vi "Fetch Cal Standard.vi"(0 "NICal5501 in":refnum<class "Cal Standard.lvclass">, 11 "error in":errorcluster) -> (4 "NICal5501 out":refnum<class "Cal Standard.lvclass">, 15 "error out":errorcluster)   [LabVIEW 2023, in "NI Cal-5501 Cal Standard.lvlib" / "Cal Standard.lvclass"]
uses:
  Cal Standard.lvclass
  C:/srd-semi-rfcal-software/AuxTools/STSRFFixtureCharactUtility/Source/Code Modules/Fixture/Instruments/Cal Standard/Cal Standard Base/Cal Standard Base.lvclass
  Cal Standard.lvclass/Cal Standard.ctl
  Instruments/Cal Standard/Type Definitions/One-Port Cal Standard.ctl
  Instruments/Cal Standard/Type Definitions/One-Port Charact Data.ctl
  Instruments/Cal Standard/Type Definitions/Standard Type.ctl
  Properties/Read Resource Name.vi
  <instrlib>/niVCalModule/niVCalUtilities.llb/vCalUtils Unpack Cal Standard Characterization Data.vi
  <instrlib>/niVCalModule/niVCalUtilities.llb/vCalUtils Cal Standard and Port to Ports.vi
  <instrlib>/niVCalModule/niVCalUtilities.llb/vCalUtils Conditionally Add Data Mismatch Error to Error Cluster.vi
  <instrlib>/niVCalModule/niVCalModule.llb/vCal Read Cal Standard Constants.vi
  <vilib>/Utility/error.llb/Error Cluster From Error Code.vi
  Instruments/Cal Standard/Cal Standard Base/Properties/Write One-Port Cal Standards.vi
  Instruments/RFFixtureCharact.Instruments.lvlib
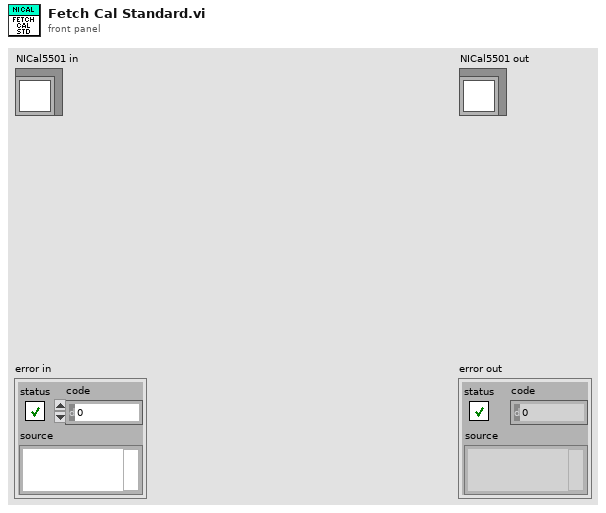
[diagram p1: front panel]
types:
  T1 = typedef "RFFixtureCharact.Instruments.lvlib/One-Port Cal Standard.ctl" = cluster{"Port Name":string, "Charact Data":T2[]}
  T2 = typedef "RFFixtureCharact.Instruments.lvlib/One-Port Charact Data.ctl" = cluster{"Standard Type":T3, "Frequencies":dbl[], "S11":cdb[]}
  T3 = typedef "RFFixtureCharact.Instruments.lvlib/Standard Type.ctl" = enum16{"Short", "Open", "Load"}
  T4 = typedef "Standard Control.ctl" = i32
  T5 = typedef "vCalUtils S Parameters (2 Port).ctl" = cluster{"S11":cluster{"frequencies":dbl[], "s parameters":cdb[]}, "S12":cluster{"frequencies":dbl[], "s parameters":cdb[]}, "S21":cluster{"frequencies":dbl[], "s parameters":cdb[]}, "S22":cluster{"frequencies":dbl[], "s parameters":cdb[]}}
  T6 = cluster{"frequencies":dbl[], "s parameters":cdb[]}
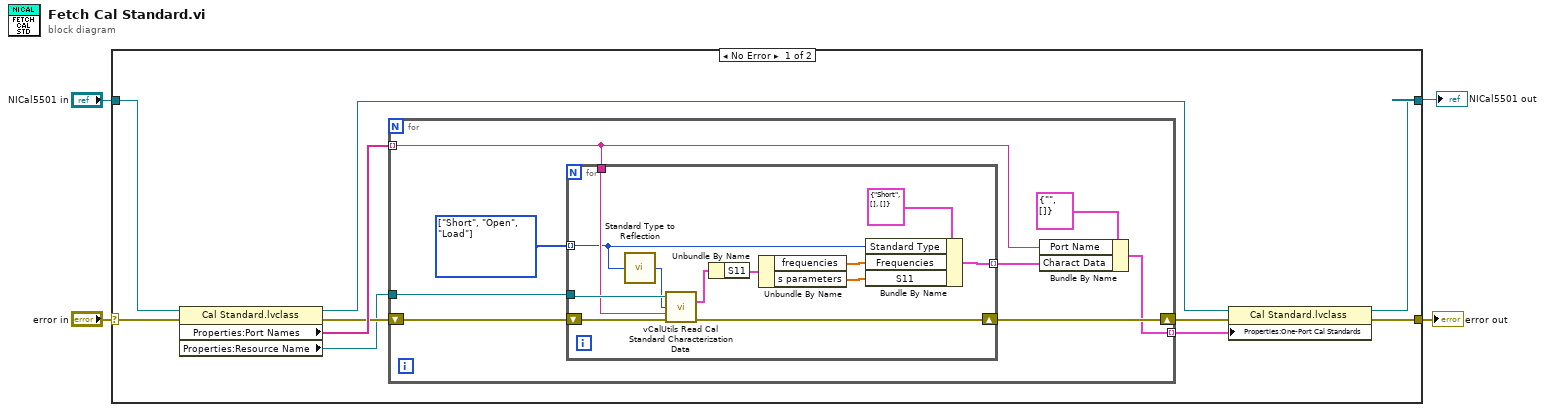
[diagram p0: block diagram]
diagram:
  n1 = case shown="No Error" "error in" {
    selector: "error in" -> [w10 w36]
    tunnel: [w13 w36] -> w2
    tunnel: [w12 w35] -> w1
    tunnel: "NICal5501 in" -> [w9 w35]
    frame No Error {
      n2 = property class="Cal Standard.lvclass"(reference=w9, error in=w10) -> (reference out=w8:refnum<class "Cal Standard.lvclass">, error out=w6:errorcluster, "Properties:Port Names"=w7:string[], "Properties:Resource Name"=w5:refnum<k15>)
      n3 = for {
        tunnel: w5 -> [w17]
        shift-right: [w22] -> w14
        shift-left: w6 -> [w16]
        tunnel: w7 -> [w19] mode=indexing
        tunnel: [w18] -> w11 mode=indexing
        w15 = T3[] [enum."Short", enum."Open", enum."Load"] items=["Short", "Open", "Load"]
        n4 = for {
          tunnel: w17 -> [w30]
          shift-right: [w31] -> w22
          shift-left: w16 -> [w32]
          tunnel: w19 -> [w29]
          tunnel: [w33] -> w20 mode=indexing
          tunnel: w15 -> [w24] mode=indexing
          n5 = call "Standard Type to Reflection.vi"("Standard Type"=w24) -> ("Standard Type"=w23:T4)
          n6 = call <instrlib>:"vCalUtils Read Cal Standard Characterization Data.vi"("vCal handle in"=w30, "calibration standard"=w23, "port"=w29, "error in"=w32) -> ("s-parameters"=w27:T5, "error out"=w31:errorcluster)  [unwired: 9 in, 1 out]
          n7 = Unbundle By Name(w27) -> ("S11"=w28:T6)
          n8 = Unbundle By Name(w28) -> ("frequencies"=w26:dbl[], "s parameters"=w25:cdb[])
          n9 = Bundle By Name(cluster=T2 {"Standard Type"=enum."Short", "Frequencies"=[], "S11"=[]} ("Cal Characterization Data"), "Standard Type"=w24, "Frequencies"=w26, "S11"=w25) -> (w33:T2)
        }
        n10 = Bundle By Name(cluster=T1 {"Port Name"="", "Charact Data"=[]} ("One-Port Cal Standard"), "Port Name"=w19, "Charact Data"=w20) -> (w18:T1)
      }
      n11 = property class="Cal Standard.lvclass"(reference=w8, error in=w14, "Properties:One-Port Cal Standards"=w11) -> (reference out=w12:refnum<class "Cal Standard.lvclass">, error out=w13:errorcluster)
    }
    frame Error {
    }
  }
  "error out" <- w2
  "NICal5501 out" <- w1
